vi "ExtractTextFromRing.vi"(8 "error in (no error)":errorcluster, 11 "Siemens Digital Energy Meter":T2 {"Measurement(s)" items=["kWh System"=4000, "kVARh System"=4007, "kVAh System"=4010, "kVA System"=4012, "Volts L1 to L2"=4018, "Volts L2 to L3"=4019, "Volts L1 to L2"=4020, "Line Frequency"=4021, "kW L1"=4028, "kW L2"=4029, "kW L3"=4030, "kVAR L1"=4037, "kVAR L2"=4038, "kVAR L3"=4039, "kVA L1"=4046, "kVA L2"=4047, "kVA L3"=4048, "Apparent PF L1"=4052, "Apparent PF L2"=4053, "Apparent PF L3"=4054, "Amps L1"=4055, "Amps L2"=4056, "Amps L3"=4057, "Volts L1 to Neutral"=4058, "Volts L2 to Neutral"=4059, "Volts L3 to Neutral"=4060, "Firmware Major Revision"=4068, "Firmware Minor Revision "=4069, "Model Number "=4200, "Serial Number"=4205, "Hardware ID"=4510]}) -> (0 "error out":errorcluster, 3 "MeasurementTypeStrings":string[][](array[string]))   [LabVIEW 2018, in "SensorPlugins.lvlib" / "SiemensDigitalEnergyMeter.lvclass"]
doc: "This VI extracts the text from the Measurements Array."
uses:
  SiemensDigitalEnergyMeter.lvclass
  TypeDefinitions/SiemensDigitalEnergyMeterControls.ctl
  <vilib>/Utility/miscctls.llb/LVStringsAndValuesArrayTypeDef.ctl
panel:
  out "Strings And Values []":T1
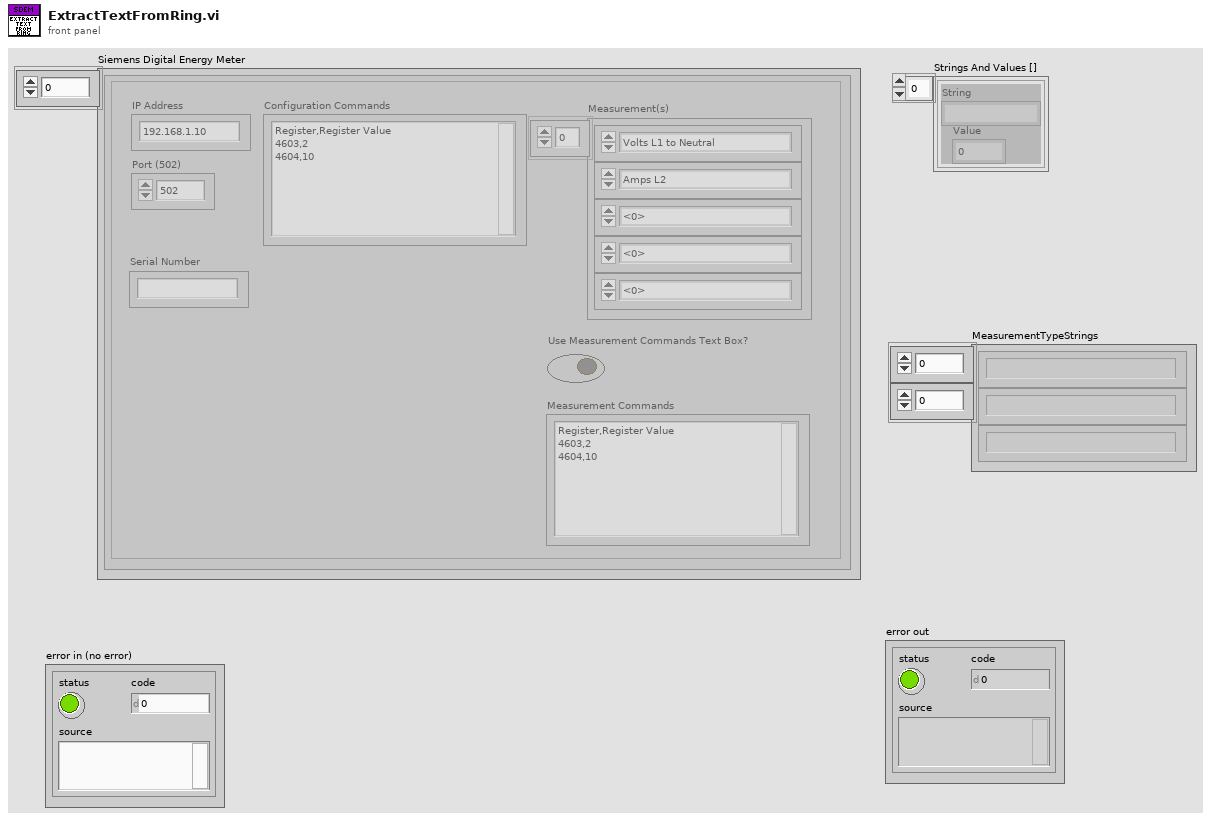
[diagram p1: front panel]
types:
  T1 = typedef "LVStringsAndValuesArrayTypeDef.ctl" = cluster{"String":string, "Value":ext}[]
  T2 = typedef "SensorPlugins.lvlib/SiemensDigitalEnergyMeter.lvclass/SiemensDigitalEnergyMeterControls.ctl" = cluster{"Measurement(s)":u16[], "IP Address":string, "Port (502)":u16, "Configuration Commands":string, "Use Measurement Commands Text Box?":bool, "Measurement Commands":string, "Connected?":bool, "Serial Number":string}[]
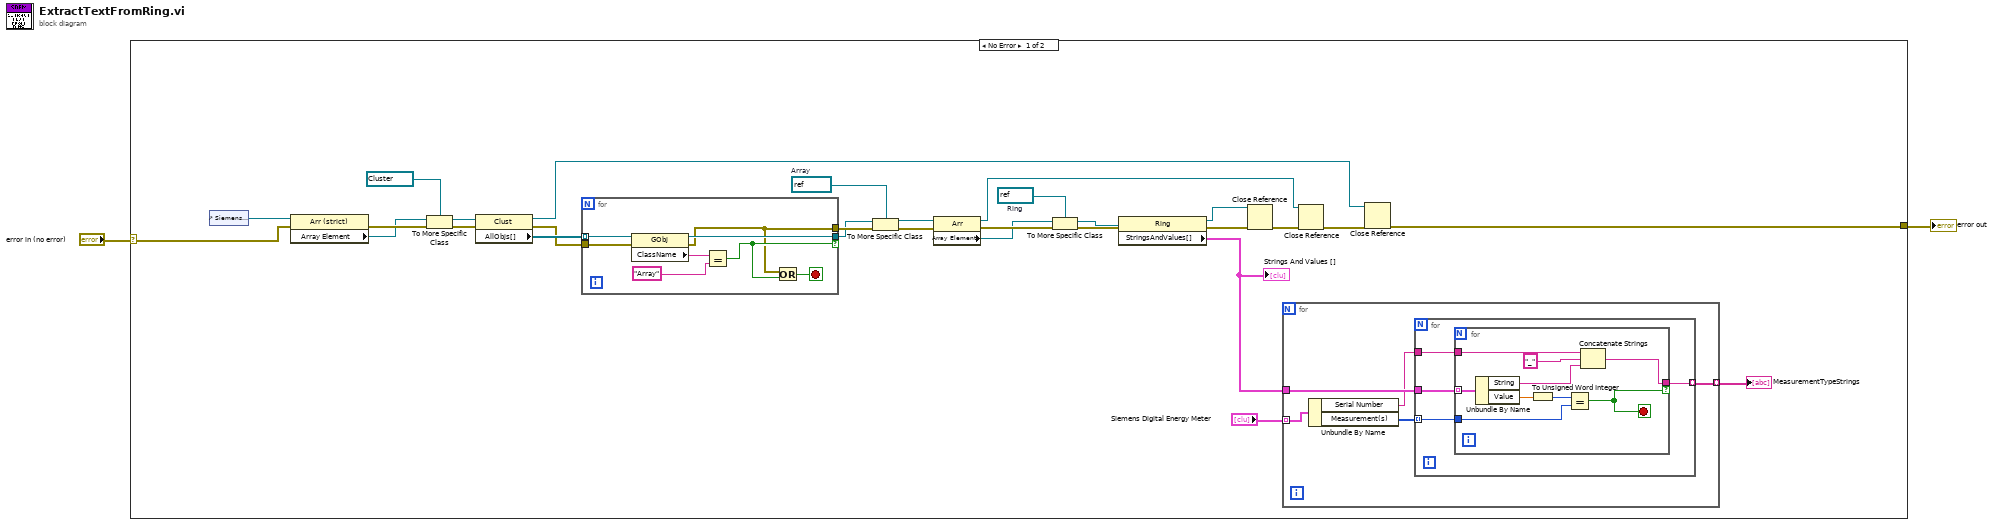
[diagram p0: block diagram]
diagram:
  n1 = case shown="No Error" "error in (no error)" {
    selector: "error in (no error)" -> [w9 w58]
    tunnel: [w8 w58] -> w1
    frame No Error {
      w23 = refnum<vi> refnum  # Ring
      w26 = refnum<vi> refnum  # Array
      n2 = control-ref of="Siemens Digital Energy Meter"() -> (w18:refnum<vi>)
      n3 = property class="Arr (strict)"(reference=w18, error in=w9) -> (error out=w31:errorcluster, "Array Element"=w30:refnum<vi>)  [unwired: 1 out]
      n4 = To More Specific Class(target class=refnum<vi> refnum ("Text Ring"), reference=w30, error in=w31) -> (specific class reference=w27:refnum<vi>, error out=w28:errorcluster)
      n5 = property class="Clust"(reference=w27, error in=w28) -> (reference out=w12:refnum<vi>, error out=w6:errorcluster, "AllObjs[]"=w7:refnum<vi>[])
      n6 = for {
        tunnel: w7 -> [w39] mode=indexing
        tunnel: [w38] -> w4 if=w33
        tunnel: w6 -> [w35]
        tunnel: [w32] -> w5
        stop <- w34 stop-if-true
        n7 = property class="GObj"(reference=w39, error in=w35) -> (reference out=w38:refnum<vi>, error out=w32:errorcluster, "ClassName"=w37:string)
        n8 = Equal?(x=w37, y="Array" ("ClassName")) -> (x = y?=w33:bool)
        n9 = Or(x=w32, y=w33) -> (x .or. y?=w34:bool)
      }
      n10 = To More Specific Class(target class=w26, reference=w4, error in=w5) -> (specific class reference=w24:refnum<vi>, error out=w25:errorcluster)
      n11 = property class="Arr"(reference=w24, error in=w25) -> (reference out=w14:refnum<vi>, error out=w22:errorcluster, "Array Element"=w21:refnum<vi>)
      n12 = To More Specific Class(target class=w23, reference=w21, error in=w22) -> (specific class reference=w19:refnum<vi>, error out=w20:errorcluster)
      n13 = property class="Ring"(reference=w19, error in=w20) -> (reference out=w16:refnum<vi>, error out=w17:errorcluster, "StringsAndValues[]"=w11:T1)
      "Strings And Values []" <- w11
      n14 = Close Reference(reference=w16, error in (no error)=w17) -> (error out=w15:errorcluster)
      n15 = for {
        tunnel: w11 -> [w44]
        tunnel: "Siemens Digital Energy Meter" -> [w43] mode=indexing
        tunnel: [w41] -> w3 mode=indexing
        n16 = Unbundle By Name(w43) -> ("Serial Number"=w40:string, "Measurement(s)"=w42:u16[])
        n17 = for {
          tunnel: w44 -> [w48]
          tunnel: w42 -> [w47] mode=indexing
          tunnel: [w46] -> w41 mode=indexing
          tunnel: w40 -> [w45]
          n18 = for {
            tunnel: w48 -> [w55] mode=indexing
            tunnel: w47 -> [w54]
            tunnel: [w51] -> w46 if=w53
            tunnel: w45 -> [w50]
            stop <- w53 stop-if-true
            n19 = Unbundle By Name(w55) -> ("String"=w52:string, "Value"=w57:ext)
            n20 = To Unsigned Word Integer(number=w57) -> (unsigned 16bit integer=w56:u16)
            n21 = Equal?(x=w56, y=w54) -> (x = y?=w53:bool)
            n22 = Concatenate Strings(w50, "_" ("string"), w52) -> (w51:string)
          }
        }
      }
      "MeasurementTypeStrings" <- w3
      n23 = Close Reference(reference=w14, error in (no error)=w15) -> (error out=w13:errorcluster)
      n24 = Close Reference(reference=w12, error in (no error)=w13) -> (error out=w8:errorcluster)
    }
    frame Error {
    }
  }
  "error out" <- w1
